vi "Configure Arbitrary Waveform.vi"(0 "RedPitaya connection in":refnum<k5>, 2 "Data":dbl[](array[numeric])=[0.0], 5 "error in":errorcluster, 8 "Channel #":u16(ring)=1 items=["Channel 1"=1, "Channel 2"=2], 12 "timeout ms (2000)":i32=2000) -> (14 "RedPitaya connection out":refnum<k5>, 19 "error out":errorcluster)   [LabVIEW 2010, in "RedPitaya.lvlib"]
doc: "Configures the arbitrary waveform generator options"
uses:
  RedPitaya.lvlib
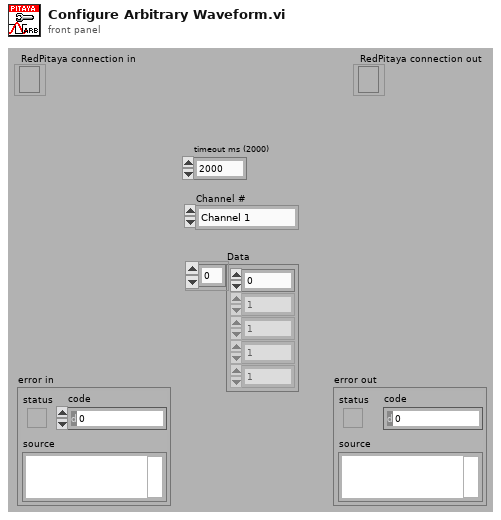
[diagram p1: front panel]
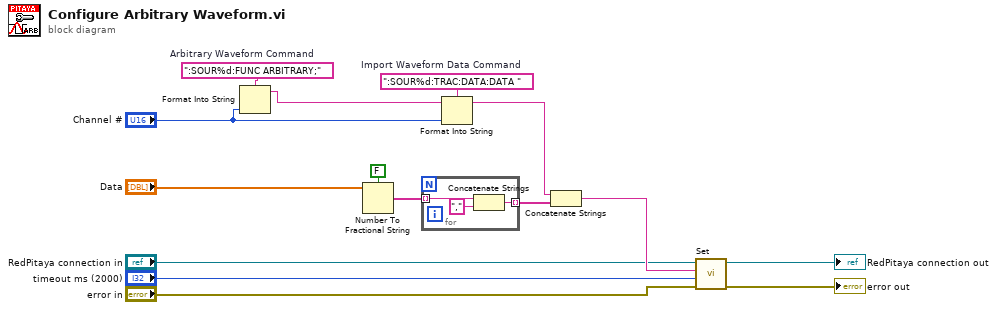
[diagram p0: block diagram]
diagram:
  w5 = ":SOUR%d:FUNC ARBITRARY;"  # Arbitrary Waveform Command
  w15 = ":SOUR%d:TRAC:DATA:DATA "  # Import Waveform Data Command
  n1 = Format Into String(format string=w5, "Channel #") -> (resulting string=w4:string)  [unwired: 2 in, 1 out]
  n2 = Number To Fractional String(use system decimal point (T)=FALSE, number="Data") -> (F-format string=w10:string[])  [unwired: 2 in]
  n3 = for {
    tunnel: w10 -> [w18] mode=indexing
    tunnel: [w16] -> w12 mode=indexing
    n4 = Concatenate Strings(w18, "," ("string")) -> (w16:string)
  }
  n5 = Format Into String(format string=w15, initial string=w4, "Channel #") -> (resulting string=w11:string)  [unwired: 1 in, 1 out]
  n6 = Concatenate Strings(w11, w12) -> (w9:string)
  n7 = call "Set.vi"("error in"="error in", "timeout ms (2000)"="timeout ms (2000)", "SCPI Message"=w9, "RedPitaya connection in"="RedPitaya connection in") -> ("error out"=→"error out":errorcluster, "RedPitaya connection out"=→"RedPitaya connection out":refnum<k5>)  [unwired: 5 in, 1 out]
